vi "ReplaceObject.vi"(6 "name/order":string="LabVIEW Object In", 8 "error in (no error)":errorcluster, 11 "CreateClass In":refnum<class "CreateClass.lvclass">) -> (0 "error out":errorcluster)   [LabVIEW 2020, in "Mermaid.lvlib" / "CreateClass.lvclass"]
uses:
  CreateClass.lvclass
  CreateClass.lvclass/CreateClass.ctl
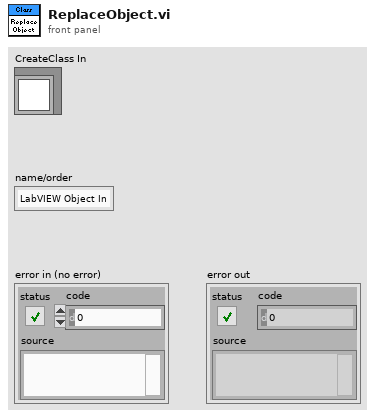
[diagram p1: front panel]
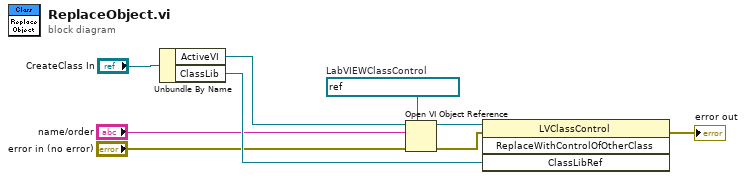
[diagram p0: block diagram]
diagram:
  w4 = refnum<vi> refnum  # LabVIEWClassControl
  n1 = Unbundle By Name("CreateClass In") -> ("ActiveVI"=w8:refnum<vi>, "ClassLib"=w9:refnum<vi>)
  n2 = Open VI Object Reference(7:w4, 8:"error in (no error)", 10:"name/order", 11:w8) -> (0:w3:errorcluster, 3:w5:refnum<vi>)
  n3 = invoke class="LVClassControl" method="ReplaceWithControlOfOtherClass"(reference=w5, error in=w3, "ClassLibRef"=w9) -> (error out=→"error out":errorcluster)  [unwired: 1 in, 3 out]
